vi "New URI.vi"(5 "URI in":refnum<class "URI.lvclass">, 8 "error in (no error)":errorcluster, 10 "base-path":string, 11 "URI":string) -> (0 "error out":errorcluster, 3 "URI":refnum<class "URI.lvclass">)   [LabVIEW 2013, in "openURI.lvlib" / "URI.lvclass"]
uses:
  URI.lvclass
  URI.lvclass/URI.ctl
  utilities/Extract URI Components.vi
  openURI.lvlib
  components/path/URI-Component.Path.lvclass
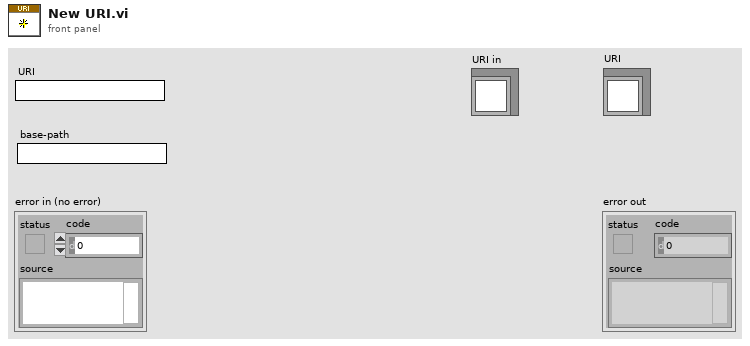
[diagram p1: front panel]
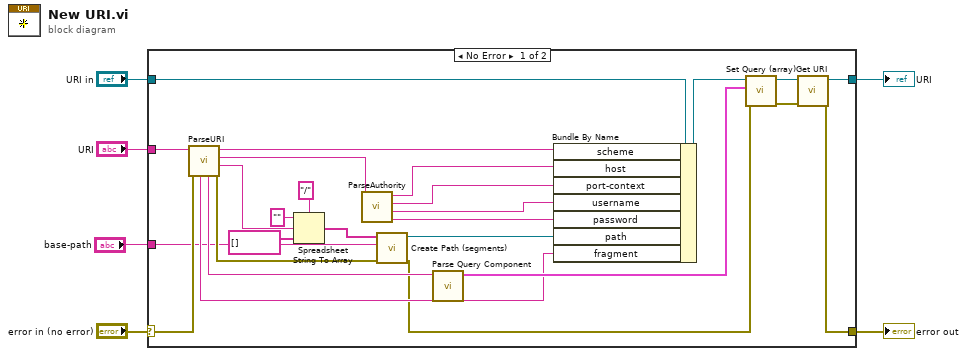
[diagram p0: block diagram]
diagram:
  n1 = case shown="No Error" "error in (no error)" {
    selector: "error in (no error)" -> [w27 w34]
    tunnel: [w21 w34] -> w5
    tunnel: [w23 w33] -> w3
    tunnel: "URI in" -> [w8 w33]
    tunnel: "URI" -> [w20 _]
    tunnel: "base-path" -> [w7 _]
    frame No Error {
      n2 = call "ParseURI.vi"("error in"=w27, "URI"=w20) -> ("error out"=w18:errorcluster, "path"=w15:string, "authority"=w32:string, "scheme"=w9:string, "query"=w28:string, "fragment"=w19:string)  [unwired: 4 in]
      n3 = Spreadsheet String To Array(delimiter (Tab)="/", format string="", spreadsheet string=w15, array type (2D Dbl)=string[] [] ("Segments")) -> (array=w13:string[])
      n4 = call "ParseAuthority.vi"("authority"=w32) -> ("password"=w29:string, "username"=w30:string, "port"=w10:string, "host"=w31:string)  [unwired: 7 in]
      n5 = call "Create Path (segments).vi"("error in (no error)"=w18, "base-path"=w7, "Segments"=w13) -> ("error out"=w17:errorcluster, "URI-Component.Path"=w16:refnum<class "URI-Component.Path.lvclass">)  [unwired: 6 in, 1 out]
      n6 = call "Parse Query Component.vi"("query"=w28) -> ("Query"=w25:cluster{"argument":string, "value":string}[])  [unwired: 10 in]
      n7 = Bundle By Name(cluster=w8, "scheme"=w9, "host"=w31, "port-context"=w10, "username"=w30, "password"=w29, "path"=w16, "fragment"=w19) -> (w26:refnum<class "URI.lvclass">)
      n8 = call "Set Query (array).vi"("error in (no error)"=w17, "Query"=w25, "URI in"=w26) -> ("error out"=w22:errorcluster, "URI out"=w24:refnum<class "URI.lvclass">)  [unwired: 7 in]
      n9 = call "Get URI.vi"("error in (no error)"=w22, "URI in"=w24) -> ("error out"=w21:errorcluster, "URI"=w23:refnum<class "URI.lvclass">)  [unwired: 7 in, 1 out]
    }
    frame Error {
    }
  }
  "error out" <- w5
  "URI" <- w3
